vi "HISW_constructor.vi"(7 "FAMM.lvclass":refnum<class "FAMM.lvclass">, 8 "error in (no error)":errorcluster, 9 "DAQ-Queue":refnum<queue>, 10 "FAMM-Queue":refnum<queue>, 11 "HISW in":refnum<class "HISW.lvclass">) -> (0 "error out":errorcluster, 3 "HISW out":refnum<class "HISW.lvclass">)   [LabVIEW 2020, in "Sgraph_lib_V1.lvlib" / "HISW.lvclass"]
uses:
  HISW.lvclass
  C:/Sgraph/Sgraph/source/FAMM/FAMM.lvclass
  C:/Sgraph/Sgraph/source/AVPP/AVPP.lvclass
  FAMM/controls/typedef_FAMM_Query.ctl
  FAMM/controls/typedef-functions.ctl
  controls/typedef-DAQ-datagram.ctl
  controls/typedef-Qtype.ctl
  FAMM/FAMM.lvclass
  HISW.lvclass/HISW.ctl
  FAMM/FAMM.lvclass/FAMM.ctl
  AVPP/AVPP.lvclass
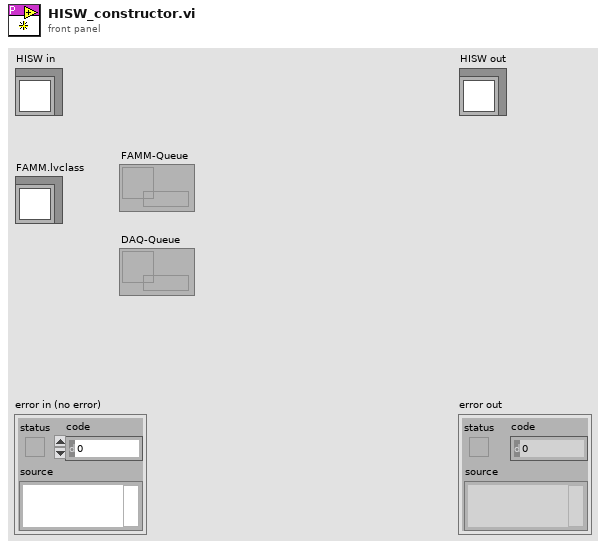
[diagram p1: front panel]
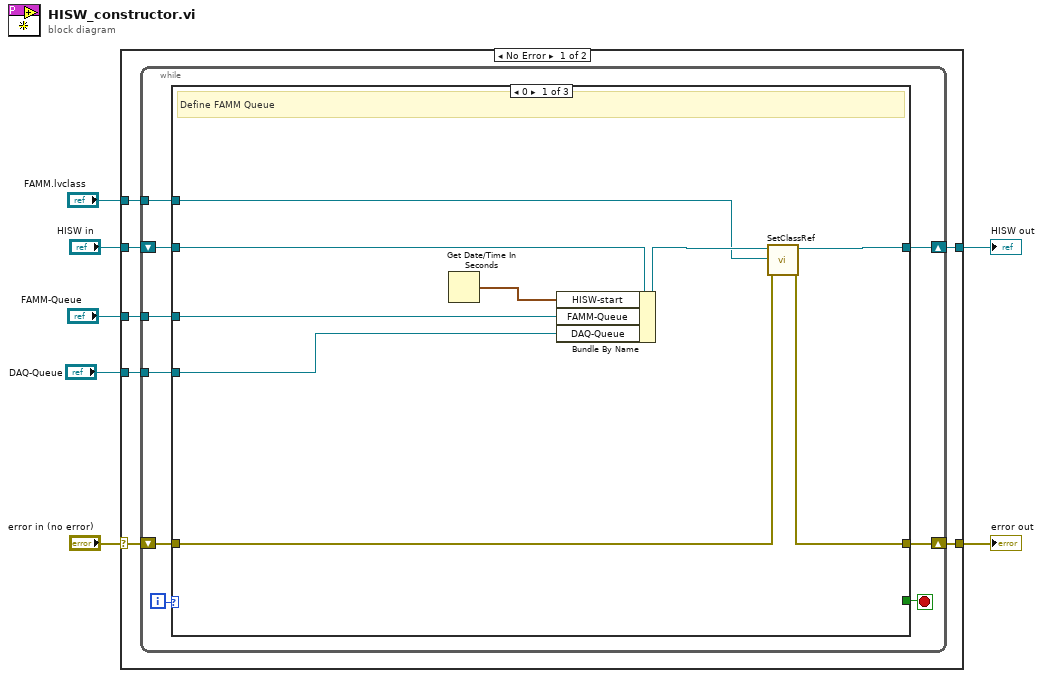
[diagram p0: block diagram]
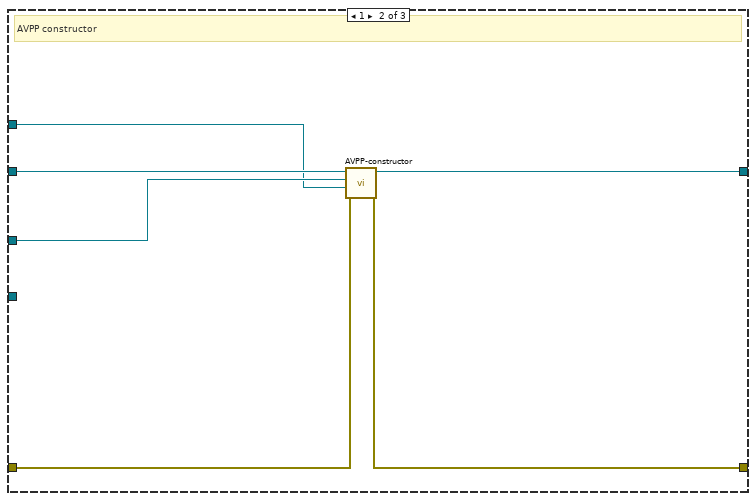
[diagram p2: hidden frame]
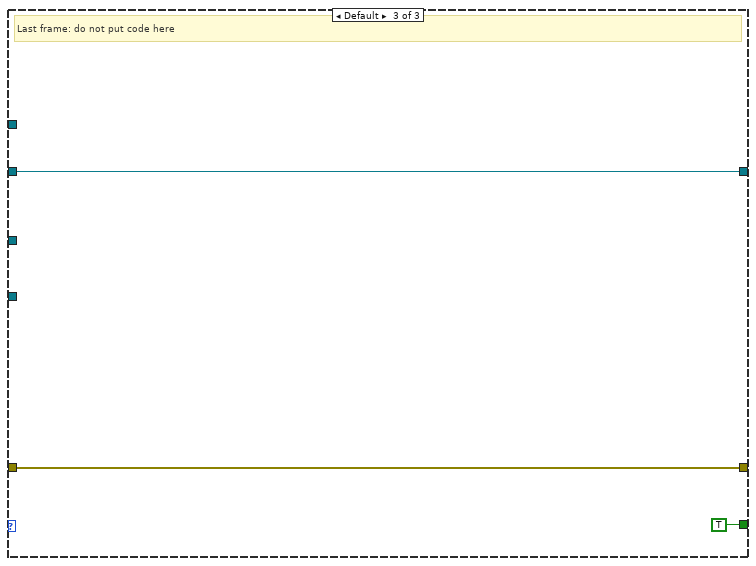
[diagram p3: hidden frame]
diagram:
  n1 = case shown="No Error" "error in (no error)" {
    selector: "error in (no error)" -> [w13 w43]
    tunnel: [w12 w43] -> w6
    tunnel: [w11 w42] -> w4
    tunnel: "HISW in" -> [w14 w42]
    tunnel: "FAMM-Queue" -> [w10 _]
    tunnel: "DAQ-Queue" -> [w9 _]
    tunnel: "FAMM.lvclass" -> [w8 _]
    frame No Error {
      n2 = while {
        shift-right: [w18] -> w12
        shift-left: w13 -> [w22]
        shift-right: [w19] -> w11
        shift-left: w14 -> [w23]
        tunnel: w10 -> [w17]
        tunnel: w9 -> [w16]
        tunnel: w8 -> [w15]
        i -> [w21]
        stop <- w20 stop-if-true
        n3 = case shown="0" w21 {
          tunnel: w23 -> [w29 w36 w39]
          tunnel: w22 -> [w24 w38 w41]
          tunnel: [_ _ TRUE] -> w20
          tunnel: [w27 w35 w39] -> w19
          tunnel: [w25 w37 w41] -> w18
          tunnel: w17 -> [w31 w34 _]
          tunnel: w16 -> [w30 _ _]
          tunnel: w15 -> [w26 w33 _]
          frame 0 {
            # "Define FAMM Queue"
            n4 = Get Date/Time In Seconds() -> (seconds since 1Jan1904=w32:timestamp)
            n5 = Bundle By Name(cluster=w29, "HISW-start"=w32, "FAMM-Queue"=w31, "DAQ-Queue"=w30) -> (w28:refnum<class "HISW.lvclass">)
            n6 = call "SetClassRef.vi"("error in (no error)"=w24, "FAMM.lvclass"=w26, "FAMM in"=w28) -> ("error out"=w25:errorcluster, "FAMM out"=w27:refnum<class "HISW.lvclass">)  [unwired: 7 in]
          }
          frame 1 {
            # "AVPP constructor"
            n7 = call "AVPP-constructor.vi"("error in (no error)"=w38, "FAMM.lvclass"=w33, "FAMM-Queue"=w34, "AVPP in"=w36) -> ("error out"=w37:errorcluster, "AVPP out"=w35:refnum<class "HISW.lvclass">)  [unwired: 6 in]
          }
          frame Default {
            # "Last frame: do not put code here"
          }
        }
      }
    }
    frame Error {
    }
  }
  "error out" <- w6
  "HISW out" <- w4
